vi "test.vi"() -> ()   [LabVIEW 2016]
panel:
  in  "Weight Matrix #":i32
  out "Array":dbl[][](array[numeric])
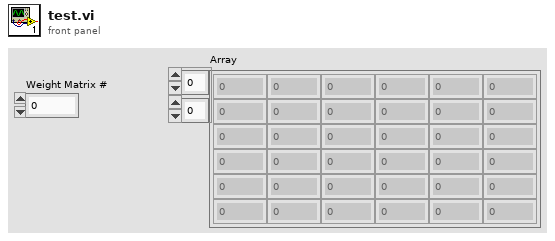
[diagram p1: front panel]
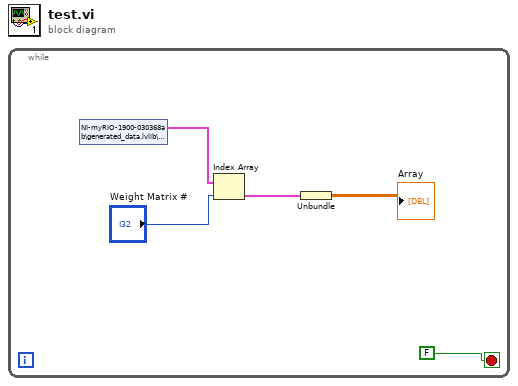
[diagram p0: block diagram]
diagram:
  n1 = while {
    stop <- FALSE stop-if-true
    n2 = shared-variable "NI-myRIO-1900-030368ab\\generated_data.lvlib\\Weights"() -> (w5:cluster{"all rows":dbl[][]}[])  [unwired: 1 in, 1 out]
    n3 = Index Array(array=w5, index="Weight Matrix #") -> (element=w2:cluster{"all rows":dbl[][]})
    n4 = Unbundle(w2) -> ("all rows"=→"Array":dbl[][])
  }
